vi "Create Macro.vi"(8 "error in (no error)":errorcluster, 9 "Macro Sequence (\"\")":string, 10 "Macro Label (\"Label\")":string="Label", 11 "VISA resource name":refnum<visa-resource-name>) -> (0 "error out":errorcluster, 3 "VISA resource name out":refnum<visa-resource-name>)   [LabVIEW 2015, in "Rohde&Schwarz CMXP Base.lvlib"]
doc: "Creates a macro. If the label exists already, the macro contents are overwritten. Macros are deleted when a remote connection is closed but can be saved to a macro file for later reuse, see MMEMory:STORe:MACRo. Avoid using labels which are identical with supported remote control commands. In contrast to SCPI stipulations, remote commands have priority over macros.\n\nAttribute:\nRSCMXPBASE_ATTR_CREATE_MACRO\n\nRemote-control command:\n*DMC"
uses:
  <instrlib>/Rohde&Schwarz CMXP Base/Rohde&Schwarz CMXP Base.lvlib
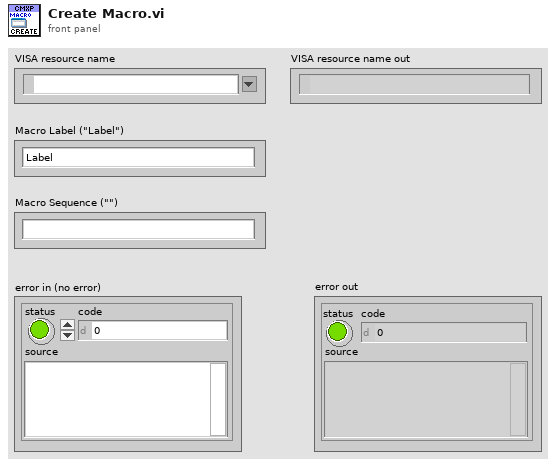
[diagram p1: front panel]
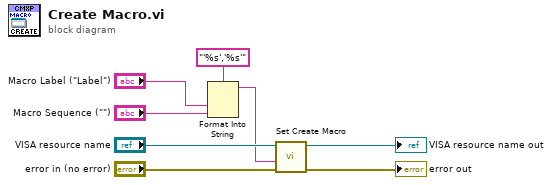
[diagram p0: block diagram]
diagram:
  n1 = Format Into String(format string="'%s','%s'", "Macro Label (\"Label\")", "Macro Sequence (\"\")") -> (resulting string=w1:string)  [unwired: 2 in, 1 out]
  n2 = call "Set Create Macro"("error in (no error)"="error in (no error)", "Create Macro ()"=w1, "instrument handle"="VISA resource name") -> ("error out"=→"error out":errorcluster, "instrument handle out"=→"VISA resource name out":refnum<visa-resource-name>)  [unwired: 7 in]
